vi "Triggers.vi"(7 "ModuleID":i32, 8 "error in (no error)":errorcluster, 10 "Triggers":T1) -> (0 "error out":errorcluster)   [LabVIEW 2014, in "FgenPlugins.lvlib" / "FgenPluginsBase.lvclass"]
uses:
  FgenPluginsBase.lvclass
  TypeDefs/clTriggers.ctl
  TypeDefs/Trigger.ctl
  TypeDefs/TriggerType.ctl
  FgenModule/Protected/clEventType.ctl
  FgenModule/FgenModule.lvlib
  FgenPlugins.lvlib
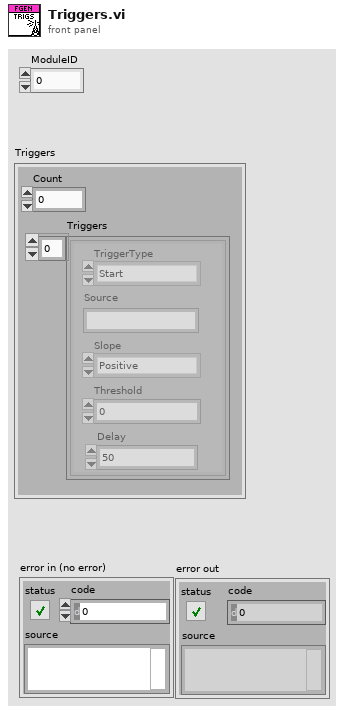
[diagram p1: front panel]
types:
  T1 = typedef "FgenPlugins.lvlib/clTriggers.ctl" = cluster{"Count":i32, "Triggers":T2[]}
  T2 = typedef "FgenPlugins.lvlib/Trigger.ctl" = cluster{"Source":string, "Slope":enum16{"Positive", "Negative", "Either"}, "Threshold":dbl, "Delay":dbl, "TriggerType":T3}
  T3 = typedef "FgenPlugins.lvlib/TriggerType.ctl" = enum16{"None", "Start", "Stop", "Hold", "Resume", "Advance"}
  T4 = typedef "FgenModule.lvlib/clEventType.ctl" = cluster{"ModuleID":i32, "Data":variant}
  T5 = typedef "FgenModule.lvlib/clBroadcastEvents.ctl" = cluster{"DidInit":refnum<user-event>, "StatusUpdate":refnum<user-event>, "ErrorReport":refnum<user-event>, "DidStop":refnum<user-event>, "PathToINI":refnum<user-event>, "Channels":refnum<user-event>, "Function":refnum<user-event>, "Waveforms":refnum<user-event>, "Triggers":refnum<user-event>}
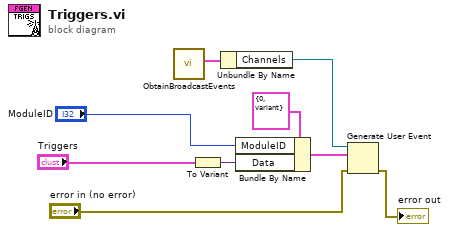
[diagram p0: block diagram]
diagram:
  n1 = call "ObtainBroadcastEvents.vi"() -> ("clBroadcastEvents"=w9:T5)  [unwired: 10 in, 1 out]
  n2 = To Variant(anything="Triggers") -> (Variant=w6:variant)
  n3 = Unbundle By Name(w9) -> ("Channels"=w8:refnum<user-event>)
  n4 = Bundle By Name(cluster=T4 {"ModuleID"=0, "Data"=variant} ("clBroadcast"), "ModuleID"="ModuleID", "Data"=w6) -> (w5:T4)
  n5 = Generate User Event(user event=w8, event data cluster=w5, error in="error in (no error)") -> (error out=→"error out":errorcluster)  [unwired: 1 in, 1 out]
